vi "胜利.vi"(1 "移动前":u16[][](array[numeric])) -> (0 "胜利？":bool)   [LabVIEW 8.6]
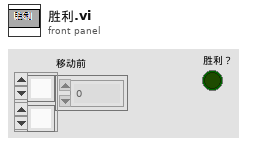
[diagram p1: front panel]
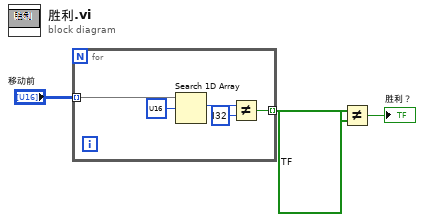
[diagram p0: block diagram]
diagram:
  n1 = for {
    tunnel: "移动前" -> [w9] mode=indexing
    tunnel: [w5] -> w3 mode=indexing
    n2 = Search 1D Array(1D array=w9, element=u16 ? ("元素")) -> (index of element=w7:i32)  [unwired: 1 in]
    n3 = Not Equal?(x=w7, y=i32 ?) -> (x != y?=w5:bool)
  }
  n4 = Not Equal?(x=w3, y=bool[] ?) -> (x != y?=→"胜利？":bool)
